vi "UpdateModTime.vi"(8 "error in (no error)":errorcluster, 10 "XML in":string, 11 "Preferences in":refnum<class "SetListPrefs.lvclass">) -> (0 "error out":errorcluster, 2 "XML out":string, 3 "Preferences out":refnum<class "SetListPrefs.lvclass">)   [LabVIEW 2013, in "SetListPrefs.lvclass"]
uses:
  SetListPrefs.lvclass
  SetListPrefs.lvclass/SetListPrefs.ctl
  <vilib>/regexp/Match Regular Expression.xnode
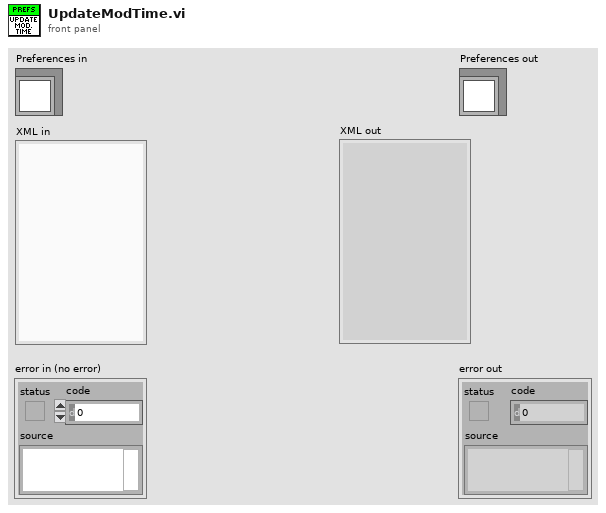
[diagram p1: front panel]
types:
  T1 = typedef "SetListPrefs.lvclass/PrefCluster.ctl" = cluster{"StartupWindowPosition":cluster{"WindowBounds":T2, "ResetPositionAtStartup":bool}, "HiddenDevices":string[], "AutoPressHWUpdate":bool, "DetachVMUIonStart":bool, "ProcRepo":path, "GitCmd":string, "GitAuths":string[][], "LoadRecentContents":string[], "SharedVariableDeployIP":string}
  T2 = typedef "LVRectTypeDef.ctl" = cluster{"Left":i16, "Top":i16, "Right":i16, "Bottom":i16}
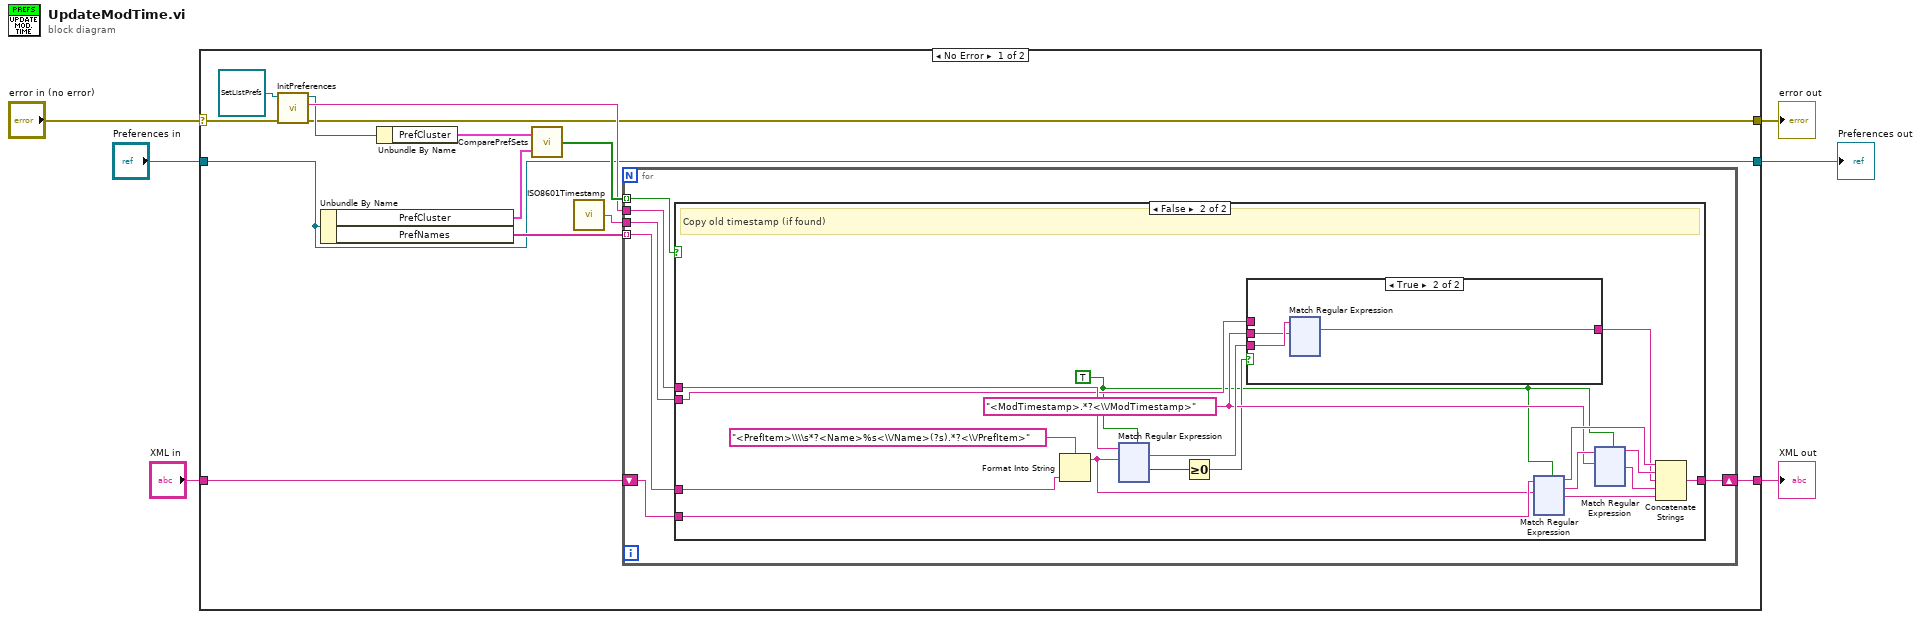
[diagram p0: block diagram]
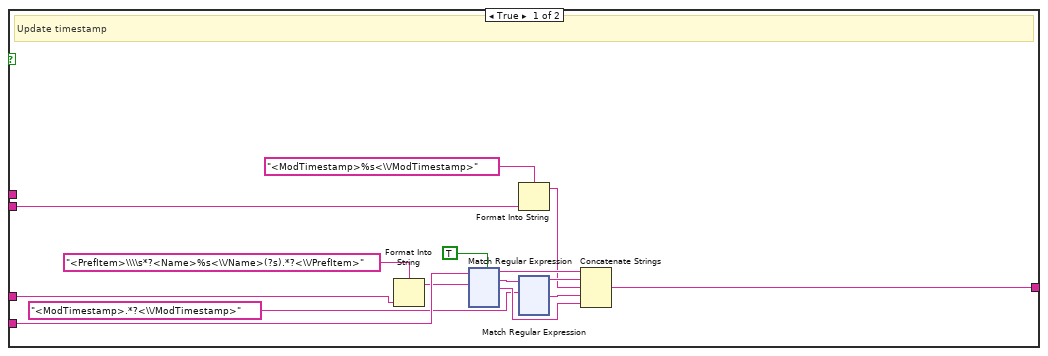
[diagram p2: hidden frame]
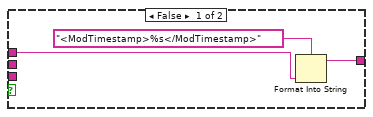
[diagram p3: hidden frame]
diagram:
  n1 = case shown="No Error" "error in (no error)" {
    selector: "error in (no error)" -> [w12 w751]
    tunnel: [w7 w751] -> w5
    tunnel: [w10 w750] -> w3
    tunnel: "Preferences in" -> [w10 w750]
    tunnel: "XML in" -> [w18 w749]
    tunnel: [w17 w749] -> w1
    frame No Error {
      n2 = call-dynamic "InitPreferences.vi"("error in (no error)"=w12, "Preferences in"=refnum<class "SetListPrefs.lvclass"> refnum ("Preferences.lvclass")) -> ("error out"=w7:errorcluster, "Raw XML"=w14:string, "Preferences out"=w8:refnum<class "SetListPrefs.lvclass">)  [unwired: 7 in]
      n3 = Unbundle By Name(w10) -> ("PrefCluster"=w11:T1, "PrefNames"=w19:string[])
      n4 = Unbundle By Name(w8) -> ("PrefCluster"=w9:T1)
      n5 = call "ComparePrefSets.vi"("Prefs B"=w11, "Prefs A"=w9) -> ("PrefDiffersArray"=w15:bool[])
      n6 = call "ISO8601Timestamp.vi"() -> ("ISO8601 Timestamp"=w16:string)
      n7 = for {
        tunnel: w15 -> [w23] mode=indexing
        tunnel: w19 -> [w21] mode=indexing
        shift-right: [w24] -> w17
        shift-left: w18 -> [w25]
        tunnel: w16 -> [w22]
        tunnel: w14 -> [w20]
        n8 = case shown="False" w23 {
          tunnel: w25 -> [w40 w286]
          tunnel: [w28 w279] -> w24
          tunnel: w22 -> [w27 w271]
          tunnel: w21 -> [w38 w285]
          tunnel: w20 -> [_ w278]
          frame True {
            # "Update timestamp"
            n9 = Format Into String(format string="<PrefItem>\\\\s*?<Name>%s<\\/Name>(?s).*?<\\/PrefItem>", w38) -> (resulting string=w37:string)  [unwired: 2 in, 1 out]
            n10 = xnode "Match Regular Expression"("input string"=w40, "regular expression"=w37, "multiline? (F)"=TRUE) -> ("before match"=w35:string, "whole match"=w36:string, "after match"=w32:string)  [unwired: 3 in, 2 out]
            n11 = Format Into String(format string="<ModTimestamp>%s<\\/ModTimestamp>", w27) -> (resulting string=w30:string)  [unwired: 2 in, 1 out]
            n12 = xnode "Match Regular Expression"("input string"=w36, "regular expression"="<ModTimestamp>.*?<\\/ModTimestamp>" ("format string")) -> ("before match"=w34:string, "after match"=w33:string)  [unwired: 4 in, 3 out]
            n13 = Concatenate Strings(w35, w34, w30, w33, w32) -> (w28:string)
          }
          frame False {
            w270 = TRUE
            w275 = "<ModTimestamp>.*?<\\/ModTimestamp>" ("format string")
            # "Copy old timestamp (if found)"
            n14 = Format Into String(format string="<PrefItem>\\\\s*?<Name>%s<\\/Name>(?s).*?<\\/PrefItem>", w285) -> (resulting string=w277:string)  [unwired: 2 in, 1 out]
            n15 = xnode "Match Regular Expression"("input string"=w278, "regular expression"=w277, "multiline? (F)"=w270) -> ("whole match"=w276:string, "offset past match"=w273:i32)  [unwired: 3 in, 3 out]
            n16 = Greater Or Equal To 0?(x=w273) -> (x >= 0?=w272:bool)
            n17 = case shown="True" w272 {
              tunnel: w276 -> [_ w292]
              tunnel: w275 -> [_ w291]
              tunnel: [w288 w290] -> w274
              tunnel: w271 -> [w287 _]
              frame False {
                n18 = Format Into String(format string="<ModTimestamp>%s</ModTimestamp>", w287) -> (resulting string=w288:string)  [unwired: 2 in, 1 out]
              }
              frame True {
                n19 = xnode "Match Regular Expression"("input string"=w292, "regular expression"=w291) -> ("whole match"=w290:string)  [unwired: 4 in, 4 out]
              }
            }
            n20 = xnode "Match Regular Expression"("input string"=w286, "regular expression"=w277, "multiline? (F)"=w270) -> ("before match"=w283:string, "whole match"=w284:string, "after match"=w280:string)  [unwired: 3 in, 2 out]
            n21 = xnode "Match Regular Expression"("input string"=w284, "regular expression"=w275, "multiline? (F)"=w270) -> ("before match"=w282:string, "after match"=w281:string)  [unwired: 3 in, 3 out]
            n22 = Concatenate Strings(w283, w282, w274, w281, w280) -> (w279:string)
          }
        }
      }
    }
    frame Error {
    }
  }
  "error out" <- w5
  "Preferences out" <- w3
  "XML out" <- w1
